vi "MU Get Nonius Track Offset Table Parameters.vi"(8 "error in (no error)":errorcluster, 11 "noniusTrackOffsetTable":cluster{"spoBase":i8, "spoN":i8[]}={"spoBase"=0, "spoN"=[0, 0, 0, 0, 0, 0, 0, 0, 0, 0, 0, 0, 0, 0, 0, 0]}) -> (0 "error out (no error)":errorcluster, 3 "noniusTrackOffsetTableParameters":cluster{"spoBase":u8, "spoN":u8[]})   [LabVIEW 2017, in "MU_3SL_interface.lvlib"]
uses:
  MU_3SL_interface.lvlib
  lib/MU_3SL_interface.dll
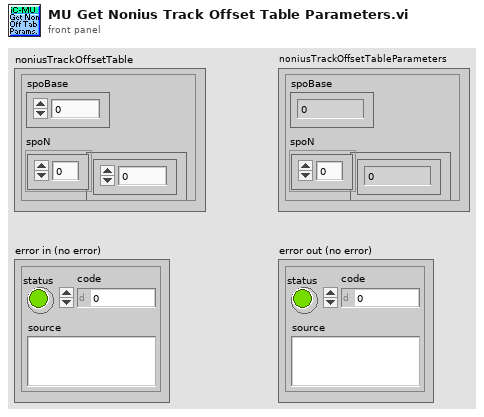
[diagram p1: front panel]
types:
  T1 = cluster{"[0]":u8, "[1]":u8, "[2]":u8, "[3]":u8, "[4]":u8, "[5]":u8, "[6]":u8, "[7]":u8, "[8]":u8, "[9]":u8, "[10]":u8, "[11]":u8, "[12]":u8, "[13]":u8, "[14]":u8, "[15]":u8}
  T2 = cluster{"[0]":i8, "[1]":i8, "[2]":i8, "[3]":i8, "[4]":i8, "[5]":i8, "[6]":i8, "[7]":i8, "[8]":i8, "[9]":i8, "[10]":i8, "[11]":i8, "[12]":i8, "[13]":i8, "[14]":i8, "[15]":i8, "[16]":i8}
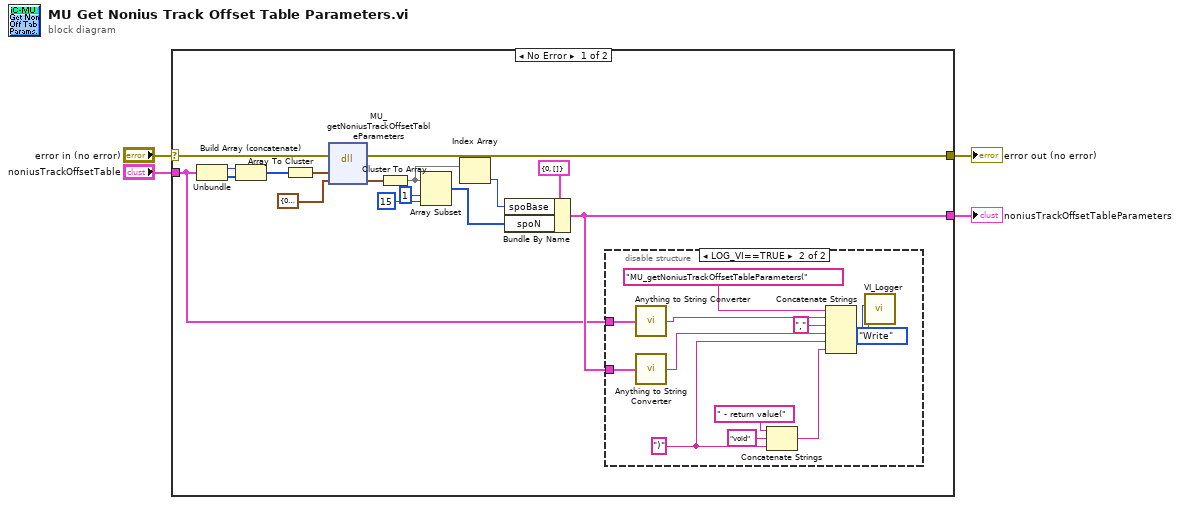
[diagram p0: block diagram]
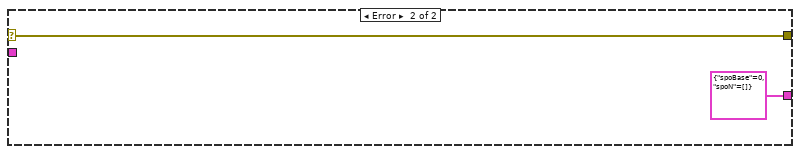
[diagram p3: hidden frame]
diagram:
  n1 = case shown="No Error" "error in (no error)" {
    selector: "error in (no error)" -> [w20 w34]
    tunnel: [w19 w34] -> w4
    tunnel: "noniusTrackOffsetTable" -> [w5 _]
    tunnel: [w11 cluster{"spoBase":u8, "spoN":u8[]} {"spoBase"=0, "spoN"=[]} ("optimizedNoniusTrackOffsetTable")] -> w1
    frame No Error {
      n2 = Unbundle(w5) -> ("spoBase"=w10:i8, "spoN"=w9:i8[])
      n3 = Build Array (concatenate)(w10, w9) -> (w8:i8[])
      n4 = Array To Cluster(array=w8) -> (cluster=w7:T2)
      n5 = dll-call lib="C:/Users/bes/AppData/Roaming/work/mu_9so/icsubmodules/soft_mu_3sl_master/lv_interface/lib/MU_3SL_interface**.*" fn="MU_getNoniusTrackOffsetTableParameters"(error in=w20, "noniusTrackOffsetTable"=w7, "noniusTrackOffsetTableParameters"=T1 {"[0]"=0, "[1]"=0, "[2]"=0, "[3]"=0, "[4]"=0, "[5]"=0, "[6]"=0, "[7]"=0, "[8]"=0, "[9]"=0, "[10]"=0, "[11]"=0, "[12]"=0, "[13]"=0, "[14]"=0, "[15]"=0} ("cluster")) -> (error out=w19:errorcluster, "noniusTrackOffsetTableParameters"=w13:T1)  [unwired: 4 in, 1 out]
      n6 = Cluster To Array(cluster=w13) -> (array=w16:u8[])
      n7 = Array Subset(array=w16, index=1, length=15) -> (w14:u8[])
      n8 = Index Array(array=w16) -> (element=w15:u8)  [unwired: 1 in]
      n9 = Bundle By Name(cluster=cluster{"spoBase":u8, "spoN":u8[]} {"spoBase"=0, "spoN"=[]} ("optimizedNoniusTrackOffsetTable"), "spoBase"=w15, "spoN"=w14) -> (w11:cluster{"spoBase":u8, "spoN":u8[]})
      n10 = disable-structure shown="LOG_VI==TRUE" {
        disable-tunnel: w11 -> [_ w27]
        disable-tunnel: w5 -> [_ w23]
        frame condition #0 {
        }
        frame condition #1 (active) {
          w26 = ")" ("string")
          n11 = call "Anything to String Converter.vi"("anything"=w23) -> ("String"=w22:string)
          n12 = call "Anything to String Converter.vi"("anything"=w27) -> ("String"=w25:string)
          n13 = Concatenate Strings(" - return value(" ("string"), "void" ("string"), w26) -> (w24:string)
          n14 = Concatenate Strings("MU_getNoniusTrackOffsetTableParameters(" ("Info in"), w22, "," ("string"), w25, w26, w24) -> (w30:string)
          n15 = call "VI_Logger.vi"("Action (Read)"=enum16{"Write", "Read"}."Write", "Info in"=w30) -> ()  [unwired: 8 in, 2 out]
        }
      }
    }
    frame Error {
    }
  }
  "error out (no error)" <- w4
  "noniusTrackOffsetTableParameters" <- w1
